vi "Quit LV if in exe.vi"(8 "error in (no error)":errorcluster) -> ()   [LabVIEW 2013, in "Utility Lib.lvlib"]
doc: "This vi will check if it has been called from an exe. If so it will quit LV."
uses:
  Utility Lib.lvlib
panel:
  out "Application:Kind":T1(ring)
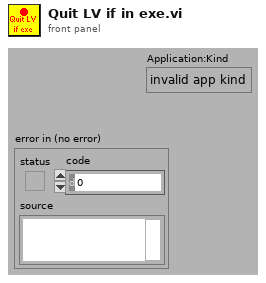
[diagram p1: front panel]
types:
  T1 = enum32{"invalid app kind", "Development System", "Run Time System", "Student Edition", "Embedded LabVIEW"}
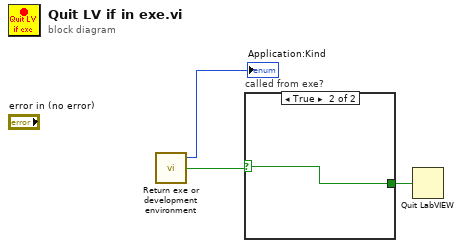
[diagram p0: block diagram]
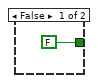
[diagram p2: hidden frame]
diagram:
  n1 = call "Return exe or development environment.vi"() -> ("exe?"=w2:bool, "Application:Kind"=→"Application:Kind":T1)  [unwired: 4 out]
  n2 = case "called from exe?" shown="True" w2 {
    selector: w2 -> [_ w5]
    tunnel: [FALSE w5] -> w3
    frame False {
    }
    frame True {
    }
  }
  n3 = Quit LabVIEW(quit? (T)=w3) -> ()
